vi "GasSettingWindow.vi"(8 "Change Param Event":refnum<user-event>, 11 "Gas parameters":T1={"Channel"=0, "RRG Gas"=1.0, "RRG expence"=0.0, "Current Gas"=0.71, "Current expence"=0.0, "description"=""} {"RRG Gas" items=["N2"=1, "SF6"=0.26, "N20"=0.71]; "Current Gas" items=["N2"=1, "SF6"=0.26, "N20"=0.71]}) -> ()   [LabVIEW 2020]
panel:
  out "Current expence":sgl
  in  "Current Gas":sgl(ring) items=["N2"=1, "SF6"=0.26, "N20"=0.71]
  in  "Close Square":bool
  in  "OK Square":bool
  in  "RRG expence":sgl
  in  "RRG Gas":sgl(ring) items=["N2"=1, "SF6"=0.26, "N20"=0.71]
  # "1. Параметры РРГ - газ"
  # "2. Параметры РРГ - max расход газа, см3"
  # "3. Подаваемый в РРГ газ"
  # "Max расход выбранного газа, см3"
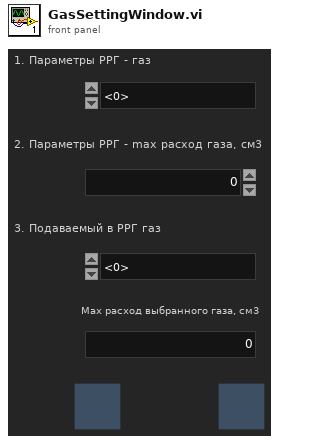
[diagram p1: front panel]
types:
  T1 = cluster{"Channel":i32, "RRG Gas":sgl, "RRG expence":sgl, "Current Gas":sgl, "Current expence":sgl, "description":string}
  T2 = enum32{"Invalid", "Standard", "Closed", "Hidden", "Minimized", "Maximized"}
  T3 = typedef "GasList.ctl" = cluster{"String":string, "Value":sgl}[]
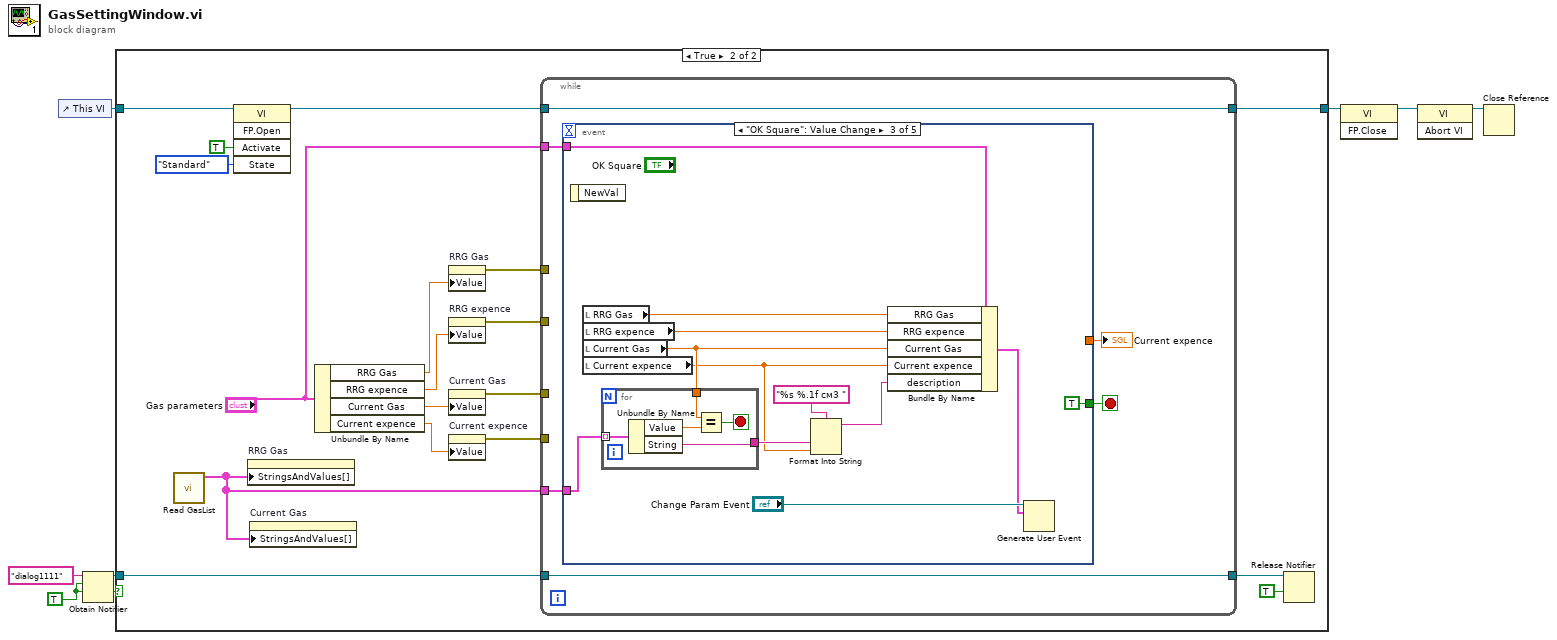
[diagram p0: block diagram]
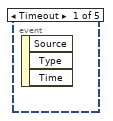
[diagram p3: hidden frame]
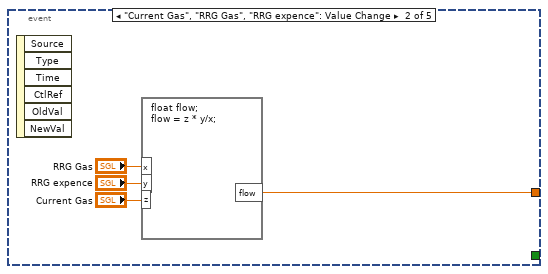
[diagram p4: hidden frame]
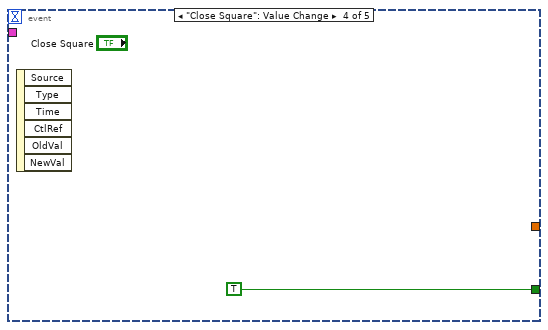
[diagram p5: hidden frame]
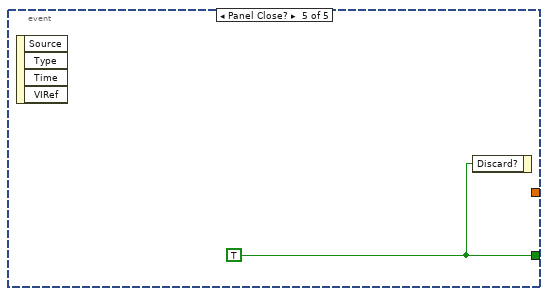
[diagram p6: hidden frame]
diagram:
  w1 = TRUE ("create if not found? (T)")
  n1 = control-ref of="This VI"() -> (w3:refnum<vi>)
  n2 = Obtain Notifier(name (unnamed)="dialog1111", notification data type=w1, create if not found? (T)=w1) -> (notifier out=w5:refnum<notifier>, created new?=w4:bool)  [unwired: 1 in, 1 out]
  n3 = case shown="True" w4 {
    tunnel: w3 -> [w9 w20]
    tunnel: [w9 w23] -> w8
    tunnel: w5 -> [_ w16]
    frame False {
    }
    frame True {
      n4 = call "Read GasList.vi"() -> ("value"=w11:T3)  [unwired: 11 in]
      n5 = invoke class="VI" method="FP.Open"(reference=w20, "Activate"=TRUE ("Activate?"), "State"=T2."Standard") -> (reference out=w19:refnum<vi>)  [unwired: 2 in, 4 out]
      n6 = property on="RRG Gas" class="Ring (strict)"("StringsAndValues[]"=w11) -> ()  [unwired: 2 in, 2 out]
      n7 = property on="Current Gas" class="Ring (strict)"("StringsAndValues[]"=w11) -> ()  [unwired: 2 in, 2 out]
      n8 = Unbundle By Name("Gas parameters") -> ("RRG Gas"=w14:sgl, "RRG expence"=w27:sgl, "Current Gas"=w12:sgl, "Current expence"=w26:sgl)
      n9 = property on="RRG Gas" class="Ring (strict)"("Value"=w14) -> (error out=w15:errorcluster)  [unwired: 2 in, 1 out]
      n10 = property on="RRG expence" class="DigNum (strict)"("Value"=w27) -> (error out=w25:errorcluster)  [unwired: 2 in, 1 out]
      n11 = property on="Current Gas" class="Ring (strict)"("Value"=w12) -> (error out=w13:errorcluster)  [unwired: 2 in, 1 out]
      n12 = property on="Current expence" class="DigNum (strict)"("Value"=w26) -> (error out=w24:errorcluster)  [unwired: 2 in, 1 out]
      n13 = while {
        tunnel: w15 -> [_]
        tunnel: w25 -> [_]
        tunnel: w13 -> [_]
        tunnel: w24 -> [_]
        tunnel: "Gas parameters" -> [w31]
        tunnel: [w30] -> w23
        tunnel: w19 -> [w30]
        tunnel: w16 -> [w29]
        tunnel: [w29] -> w22
        tunnel: w11 -> [w28]
        stop <- w32 stop-if-true
        n14 = event shown="[2] \"OK Square\": Value Change" {
          selector: _ -> [_ _ _ _ _]
          dyn-events: _ -> [_ _ _ _ _]
          timeout: _ -> [_ _ _ _ _]
          tunnel: [_ w37 _ _ _] -> w33
          tunnel: [_ _ TRUE TRUE w56] -> w32
          tunnel: w31 -> [_ _ w48 _ _]
          tunnel: w28 -> [_ _ w45 _ _]
          event Timeout {
            n15 = event-data() -> ()  [unwired: 1 in, 3 out]
          }
          event "Current Gas", "RRG Gas", "RRG expence": Value Change {
            n16 = event-data() -> ()  [unwired: 1 in, 6 out]
            n17 = formula code="float flow;\nflow = z * y/x;"("x"="RRG Gas", "y"="RRG expence", "z"="Current Gas") -> ("flow"=w37:dbl)
          }
          event "OK Square": Value Change {
            n18 = event-data() -> ()  [unwired: 1 in, 1 out]
            n19 = local read "RRG Gas"() -> (w47:sgl)
            n20 = local read "RRG expence"() -> (w46:sgl)
            n21 = local read "Current Gas"() -> (w43:sgl)
            n22 = local read "Current expence"() -> (w41:sgl)
            n23 = for {
              tunnel: w45 -> [w54] mode=indexing
              tunnel: w43 -> [w52]
              tunnel: [w50] -> w42
              stop <- w51 stop-if-true
              n24 = Unbundle By Name(w54) -> ("Value"=w53:sgl, "String"=w50:string)
              n25 = Equal?(x=w52, y=w53) -> (x = y?=w51:bool)
            }
            n26 = Format Into String(format string="%s %.1f cм3 ", w42, w41) -> (resulting string=w40:string)  [unwired: 2 in, 1 out]
            n27 = Bundle By Name(cluster=w48, "RRG Gas"=w47, "RRG expence"=w46, "Current Gas"=w43, "Current expence"=w41, "description"=w40) -> (w38:T1)
            n28 = Generate User Event(user event="Change Param Event", event data cluster=w38) -> ()  [unwired: 2 in, 2 out]
          }
          event "Close Square": Value Change {
            n29 = event-data() -> ()  [unwired: 1 in, 6 out]
          }
          event Panel Close? {
            w56 = TRUE
            n30 = event-data() -> ()  [unwired: 1 in, 4 out]
            n31 = event-data("Discard?"=w56) -> ()  [unwired: 1 in, 1 out]
          }
        }
        "Current expence" <- w33
      }
      n32 = Release Notifier(notifier=w22, force destroy? (F)=TRUE) -> ()  [unwired: 1 in, 3 out]
    }
  }
  n33 = invoke class="VI" method="FP.Close"(reference=w8) -> (reference out=w7:refnum<vi>)  [unwired: 2 in, 2 out]
  n34 = invoke class="VI" method="Abort VI"(reference=w7) -> (reference out=w6:refnum<vi>)  [unwired: 2 in, 2 out]
  n35 = Close Reference(reference=w6) -> ()  [unwired: 1 in, 1 out]
